vi "Act System PC.vi"   [LabVIEW 2014]
uses:
  <vilib>/Utility/inputDevices.llb/keyboardAcquire.vi
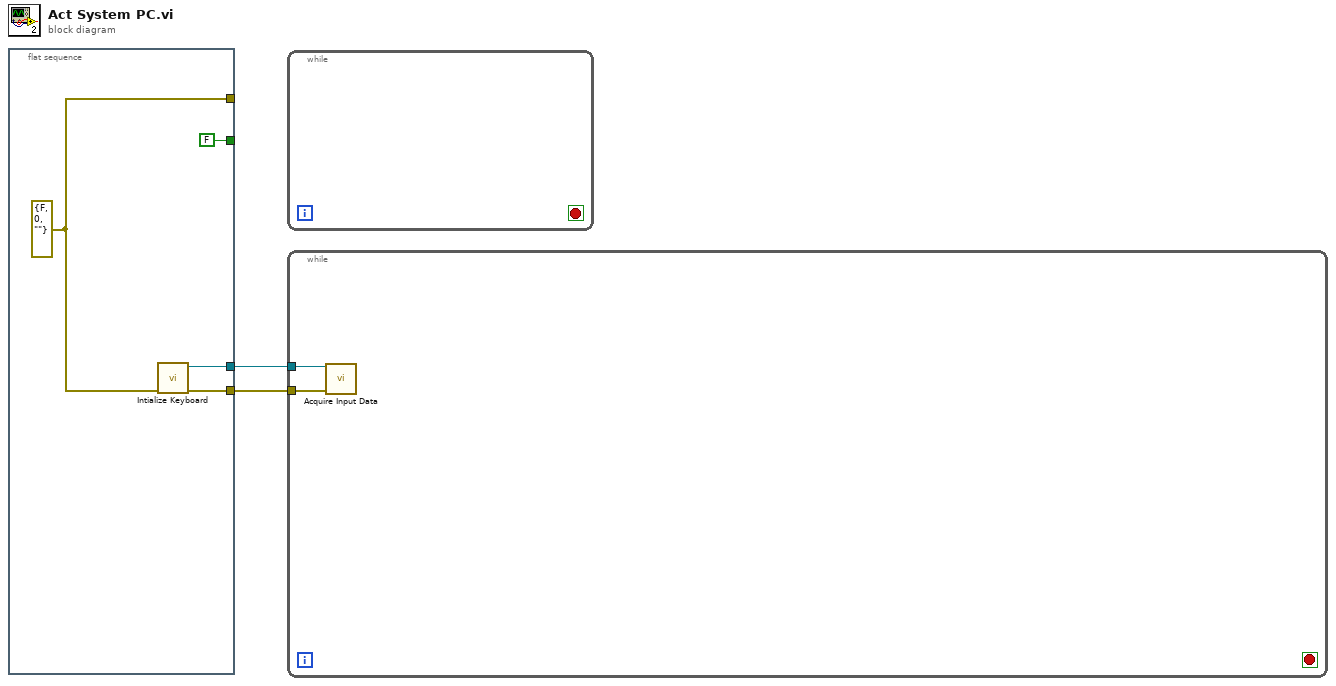
[diagram p0: block diagram]
diagram:
  n1 = flat-sequence {
    tunnel: [w6] -> _
    tunnel: [w5] -> w2
    tunnel: [w4] -> w1
    tunnel: [FALSE] -> _
    frame #0 {
      w6 = errorcluster {"status"=FALSE, "code"=0, "source"=""} ("error constant")
      n2 = call <vilib>:"Intialize Keyboard.vi"("error in (no error)"=w6) -> ("error out"=w5:errorcluster, "device ID"=w4:refnum<k1>)  [unwired: 9 in]
    }
  }
  n3 = while {
    stop <- _ stop-if-true
  }
  n4 = while {
    tunnel: w2 -> [w8]
    tunnel: w1 -> [w7]
    stop <- _ stop-if-true
    n5 = call-poly <vilib>:"Acquire Input Data.vi"("device ID"=w7, "error in (no error)"=w8) -> ()  [unwired: 15 in, 3 out]
  }
